vi "Get Tunnel Reference by Type.vi"(8 "error IO":errorcluster, 9 "Input Tunnel (F)/Output Tunnel (T)":bool, 10 "Tunnel Type":variant, 11 "Case Refnum In":refnum<vi>) -> (0 "error out":errorcluster, 1 "Desired Tunnel Reference":refnum<vi>, 3 "Case Refnum Out":refnum<vi>)   [LabVIEW 2012, in "Scripting Tools.lvlib"]
uses:
  Scripting Tools.lvlib
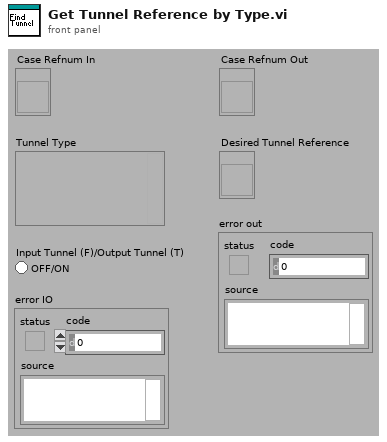
[diagram p1: front panel]
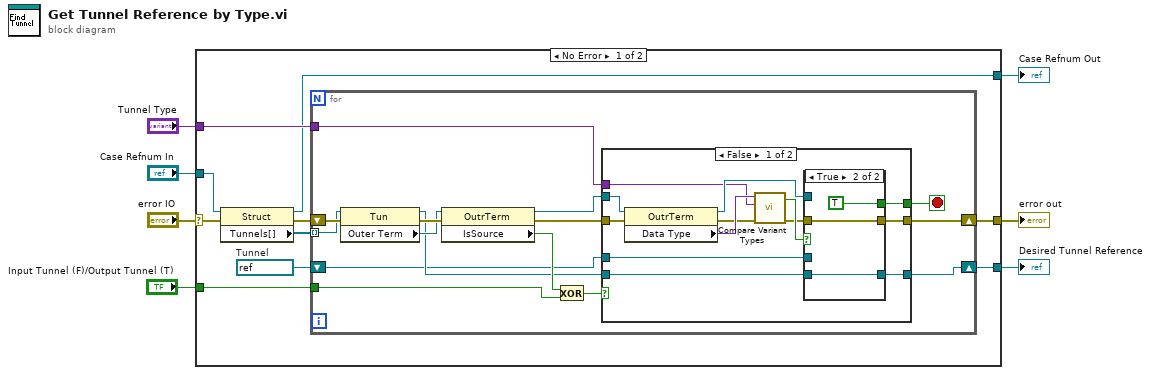
[diagram p0: block diagram]
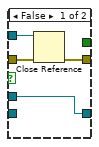
[diagram p2: hidden frame]
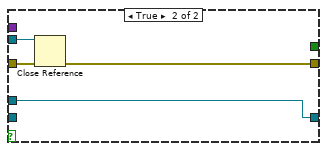
[diagram p3: hidden frame]
diagram:
  n1 = case shown="No Error" "error IO" {
    selector: "error IO" -> [w8 w57]
    tunnel: [w17 _] -> w7
    tunnel: [w16 w57] -> w6
    tunnel: "Input Tunnel (F)/Output Tunnel (T)" -> [w15 _]
    tunnel: "Tunnel Type" -> [w14 _]
    tunnel: [w13 _] -> w2
    tunnel: "Case Refnum In" -> [w9 _]
    frame No Error {
      w12 = refnum<vi> refnum  # Tunnel
      n2 = property class="Struct"(reference=w9, error in=w8) -> (reference out=w13:refnum<vi>, error out=w10:errorcluster, "Tunnels[]"=w11:refnum<vi>[])
      n3 = for {
        shift-right: [w22] -> w16
        shift-left: w10 -> [w32]
        tunnel: w11 -> [w31] mode=indexing
        shift-right: [w26] -> w17
        shift-left: w12 -> [w23]
        tunnel: w14 -> [w21]
        tunnel: w15 -> [w19]
        stop <- w18 stop-if-true
        n4 = property class="Tun"(reference=w31, error in=w32) -> (reference out=w24:refnum<vi>, error out=w30:errorcluster, "Outer Term"=w25:refnum<vi>)
        n5 = property class="OutrTerm"(reference=w25, error in=w30) -> (reference out=w28:refnum<vi>, error out=w27:errorcluster, "IsSource"=w29:bool)
        n6 = Exclusive Or(1:w19, 2:w29) -> (0:w20:bool)
        n7 = case shown="False" w20 {
          tunnel: w28 -> [w44 w55]
          tunnel: w27 -> [w45 w54]
          tunnel: [w42 w56] -> w26
          tunnel: w24 -> [w41 _]
          tunnel: w23 -> [w40 w56]
          tunnel: [w39 w53] -> w22
          tunnel: w21 -> [w36 _]
          tunnel: [w38 _] -> w18
          frame False {
            n8 = property class="OutrTerm"(reference=w44, error in=w45) -> (reference out=w43:refnum<vi>, error out=w34:errorcluster, "Data Type"=w37:variant)
            n9 = call "Compare Variant Types.vi"("error in (no error)"=w34, "Variant 2"=w36, "Variant"=w37) -> ("error out"=w33:errorcluster, "Variants have compatible types ?"=w35:bool)  [unwired: 7 out]
            n10 = case shown="True" w35 {
              tunnel: w43 -> [w48 _]
              tunnel: [w49 w52] -> w42
              tunnel: w41 -> [_ w52]
              tunnel: w40 -> [w49 _]
              tunnel: w33 -> [w47 w51]
              tunnel: [w46 w51] -> w39
              tunnel: [_ TRUE] -> w38
              frame False {
                n11 = Close Reference(reference=w48, error in (no error)=w47) -> (error out=w46:errorcluster)
              }
              frame True {
              }
            }
          }
          frame True {
            n12 = Close Reference(reference=w55, error in (no error)=w54) -> (error out=w53:errorcluster)
          }
        }
      }
    }
    frame Error {
    }
  }
  "Desired Tunnel Reference" <- w7
  "error out" <- w6
  "Case Refnum Out" <- w2
